vi "Read Dashboard Variables.vi"() -> ()   [LabVIEW 2020]
uses:
  <vilib>/Rock Robotics/Network Tables/NT Read Number.vi
  Framework/Robot Global Data.vi
  <vilib>/Rock Robotics/Network Tables/NT Read String.vi
panel:
  out "Pivot Duration":dbl
  out "Pivot Right Speed":dbl
  out "Pivot Left Speed":dbl
  out "Transfer Release Duration":dbl
  out "Transfer Up Duration":dbl
  out "Intake Duration":dbl
  out "Shooter Duration":dbl
  out "Transfer Release Setpoint":dbl
  out "Transfer Up Setpoint":dbl
  out "Intake Setpoint":dbl
  out "Shooter Setpoint":dbl
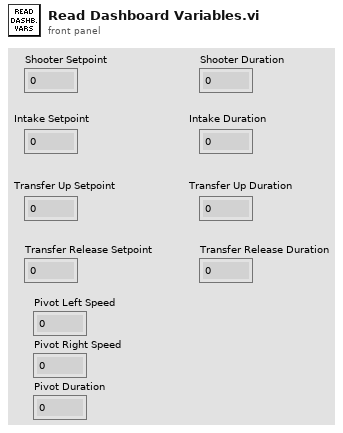
[diagram p1: front panel]
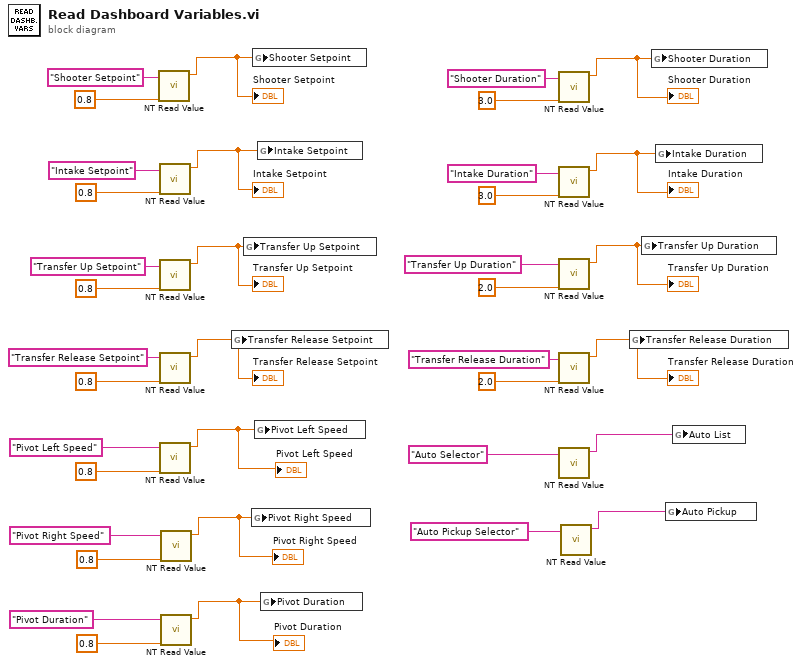
[diagram p0: block diagram]
diagram:
  n1 = call-poly <vilib>:"NT Read Value.vi"("Default Value"=0.8, "Name"="Shooter Setpoint") -> ("Numeric"=w35:dbl)  [unwired: 8 in, 1 out]
  "Shooter Setpoint" <- w35
  n2 = call-poly <vilib>:"NT Read Value.vi"("Default Value"=0.8, "Name"="Intake Setpoint") -> ("Numeric"=w20:dbl)  [unwired: 8 in, 1 out]
  "Intake Setpoint" <- w20
  n3 = call-poly <vilib>:"NT Read Value.vi"("Default Value"=0.8, "Name"="Transfer Up Setpoint") -> ("Numeric"=w19:dbl)  [unwired: 8 in, 1 out]
  "Transfer Up Setpoint" <- w19
  n4 = call-poly <vilib>:"NT Read Value.vi"("Default Value"=0.8, "Name"="Transfer Release Setpoint") -> ("Numeric"=w18:dbl)  [unwired: 8 in, 1 out]
  "Transfer Release Setpoint" <- w18
  n5 = call-poly <vilib>:"NT Read Value.vi"("Default Value"=0.8, "Name"="Pivot Left Speed") -> ("Numeric"=w7:dbl)  [unwired: 8 in, 1 out]
  "Pivot Left Speed" <- w7
  n6 = call-poly <vilib>:"NT Read Value.vi"("Default Value"=0.8, "Name"="Pivot Right Speed") -> ("Numeric"=w6:dbl)  [unwired: 8 in, 1 out]
  "Pivot Right Speed" <- w6
  n7 = call-poly <vilib>:"NT Read Value.vi"("Default Value"=0.8, "Name"="Pivot Duration") -> ("Numeric"=w5:dbl)  [unwired: 8 in, 1 out]
  "Pivot Duration" <- w5
  n8 = global write "Robot Global Data.vi" "Transfer Release Setpoint"(w18) -> ()
  n9 = global write "Robot Global Data.vi" "Transfer Up Setpoint"(w19) -> ()
  n10 = global write "Robot Global Data.vi" "Pivot Right Speed"(w6) -> ()
  n11 = global write "Robot Global Data.vi" "Shooter Setpoint"(w35) -> ()
  n12 = global write "Robot Global Data.vi" "Pivot Left Speed"(w7) -> ()
  n13 = global write "Robot Global Data.vi" "Intake Setpoint"(w20) -> ()
  n14 = global write "Robot Global Data.vi" "Pivot Duration"(w5) -> ()
  n15 = call-poly <vilib>:"NT Read Value.vi"("Default Value"=3.0, "Name"="Shooter Duration") -> ("Numeric"=w14:dbl)  [unwired: 8 in, 1 out]
  "Shooter Duration" <- w14
  n16 = call-poly <vilib>:"NT Read Value.vi"("Default Value"=3.0, "Name"="Intake Duration") -> ("Numeric"=w15:dbl)  [unwired: 8 in, 1 out]
  "Intake Duration" <- w15
  n17 = call-poly <vilib>:"NT Read Value.vi"("Default Value"=2.0, "Name"="Transfer Up Duration") -> ("Numeric"=w16:dbl)  [unwired: 8 in, 1 out]
  "Transfer Up Duration" <- w16
  n18 = call-poly <vilib>:"NT Read Value.vi"("Default Value"=2.0, "Name"="Transfer Release Duration") -> ("Numeric"=w17:dbl)  [unwired: 8 in, 1 out]
  "Transfer Release Duration" <- w17
  n19 = call-poly <vilib>:"NT Read Value.vi"("Name"="Auto Selector") -> ("String"=w4:string)  [unwired: 9 in, 1 out]
  n20 = call-poly <vilib>:"NT Read Value.vi"("Name"="Auto Pickup Selector") -> ("String"=w1:string)  [unwired: 9 in, 1 out]
  n21 = global write "Robot Global Data.vi" "Transfer Release Duration"(w17) -> ()
  n22 = global write "Robot Global Data.vi" "Transfer Up Duration"(w16) -> ()
  n23 = global write "Robot Global Data.vi" "Shooter Duration"(w14) -> ()
  n24 = global write "Robot Global Data.vi" "Intake Duration"(w15) -> ()
  n25 = global write "Robot Global Data.vi" "Auto Pickup"(w1) -> ()
  n26 = global write "Robot Global Data.vi" "Auto List"(w4) -> ()
